vi "Get Run for Execution.vi"(8 "error in (no error)":errorcluster, 11 "Schedule Cell in":refnum<class "Schedule Cell.lvclass">) -> (0 "error out":errorcluster, 1 "Last Script":bool, 2 "Run Instance":refnum<class "Run Instance.lvclass">, 3 "Schedule Cell out":refnum<class "Schedule Cell.lvclass">)   [LabVIEW 2020, in "TALOS.lvlib" / "Run Utilities.lvlib" / "Schedule Cell.lvclass"]
doc: "Get Run Instance from the Cell and change the status of the Cell to active. This VI is for manipulating Runs from the Schedule and shouldn't be used just to access the Run Instance. For obtaining Run Instance use the Read functions from Accessors or through the property node"
uses:
  Schedule Cell.lvclass
  Run Instance/Run Instance.lvclass
  Schedule Cell.lvclass/Schedule Cell.ctl
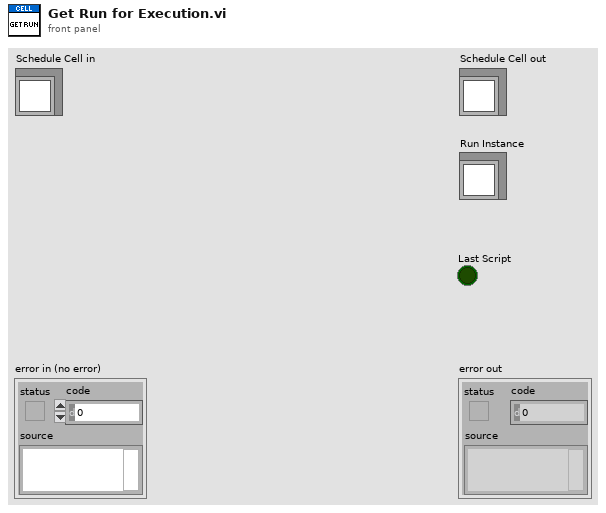
[diagram p1: front panel]
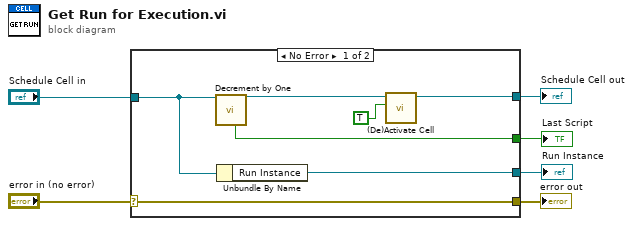
[diagram p0: block diagram]
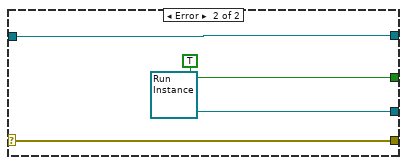
[diagram p2: hidden frame]
diagram:
  n1 = case shown="No Error" "error in (no error)" {
    selector: "error in (no error)" -> [w13 w17]
    tunnel: [w13 w17] -> w5
    tunnel: [w8 w16] -> w3
    tunnel: "Schedule Cell in" -> [w11 w16]
    tunnel: [w12 refnum<class "Run Instance.lvclass"> refnum ("Run Instance")] -> w2
    tunnel: [w10 TRUE ("Last Script")] -> w1
    frame No Error {
      n2 = call-dynamic "Decrement by One.vi"("Schedule Cell in"=w11) -> ("Schedule Cell out"=w9:refnum<class "Schedule Cell.lvclass">, "Last Script"=w10:bool)  [unwired: 7 in]
      n3 = Unbundle By Name(w11) -> ("Run Instance"=w12:refnum<class "Run Instance.lvclass">)
      n4 = call-dynamic "(De)Activate Cell.vi"("Active"=TRUE, "Schedule Cell in"=w9) -> ("Schedule Cell out"=w8:refnum<class "Schedule Cell.lvclass">)  [unwired: 8 in, 1 out]
    }
    frame Error {
    }
  }
  "error out" <- w5
  "Schedule Cell out" <- w3
  "Run Instance" <- w2
  "Last Script" <- w1
